vi "Set_Pulse.vi"(2 "error in":errorcluster, 3 "Data in":T1) -> (0 "error out":errorcluster, 1 "Data out":T1)   [LabVIEW 2017, in "Steps.lvlib"]
uses:
  Steps.lvlib
  Type_Defs/Data.ctl
  Type_Defs/Diagnostics.ctl
  Type_Defs/Systems.ctl
panel:
  in  "Helical Current":dbl[](array[numeric])
  in  "Toroidal Current":dbl[](array[numeric])
  in  "Time":dbl[](array[numeric])
  in  "Step Back":bool
  in  "Continue":bool
  # "Set the pulse for the next shot. Set the actual current that you want."
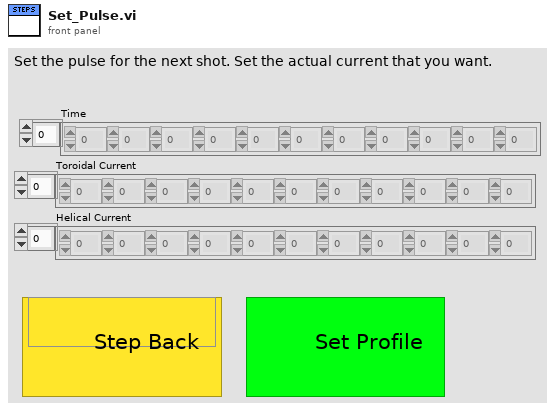
[diagram p1: front panel]
types:
  T1 = typedef "Data.ctl" = cluster{"User Name":string, "Experiment Number":i32, "Start Time":timestamp, "Data":dbl[], "Step Number":i32, "Step Instructions":string, "Diagnostics":T2, "Experiment Purpose":string, "Experiment State":enum16{"Off", "Setting Up", "Ready", "In Progress", "Shutting Down"}, "Systems":T3, "Vacuum Pressure":dbl, "Fieldpoints":cluster{"System Boolean Fieldpoints":cluster{"Compressed Air":refnum<k21>, "T-20kV Power Switch":refnum<k21>, "T-Rectifier":refnum<k21>, "Engage Interlock":refnum<k21>, "Ventilator":refnum<k21>, "Magnetron":refnum<k21>, "H-20kV Power Switch":refnum<k21>, "H-Rectifier":refnum<k21>, "Main Water Pump":refnum<k21>, "WEGA Water Pump":refnum<k21>, "Gas Inlet Valves":refnum<k21>}, "Step Fieldpoints":cluster{"Exhaust Ventillator":refnum<k21>, "Compressed Air":refnum<k21>, "Water Pressure":refnum<k21>, "Interlock":refnum<k21>, "Toroidal Power Supply 1":refnum<k21>, "Toroidal Power Supply 2":refnum<k21>, "Toroidal Rectifier":refnum<k21>, "Helical Power Supply":refnum<k21>, "Helical Rectifier":refnum<k21>, "6kW Magnetron Standby":refnum<k21>, "20kW Magnetron Standby":refnum<k21>}}, "Pressure History":cluster{"Seconds into Experiment":i32[], "Pressure Data":dbl[]}, "Time Computer Control":dbl[], "Toroidal Voltage Computer Control":dbl[], "Helical Voltage Computer Control":dbl[], "Toroidal Current":dbl[], "Toroidal Voltage":dbl[], "Toroidal Current Set Point":dbl[], "Helical Current Set Point":dbl[], "Helical Voltage":dbl[], "Helical Current":dbl[], "Experiment Folder":path, "Run Another Shot?":bool}
  T2 = typedef "Diagnostics.ctl" = cluster{"Langmuir Probe":bool, "Rogowski 1":bool, "Rogowski 2":bool, "Rogowski 3":bool, "B-dot 1":bool, "B-dot 2":bool}
  T3 = typedef "Systems.ctl" = cluster{"Compressed Air":bool, "T-20kV Power Switch":bool, "T-Rectifier":bool, "Engage Interlock":bool, "Ventilator":bool, "Magnetron":bool, "H-20kV Power Switch":bool, "H-Rectifier":bool, "Main Water Pump":bool, "WEGA Water Pump":bool, "Gas Inlet Valves":bool}
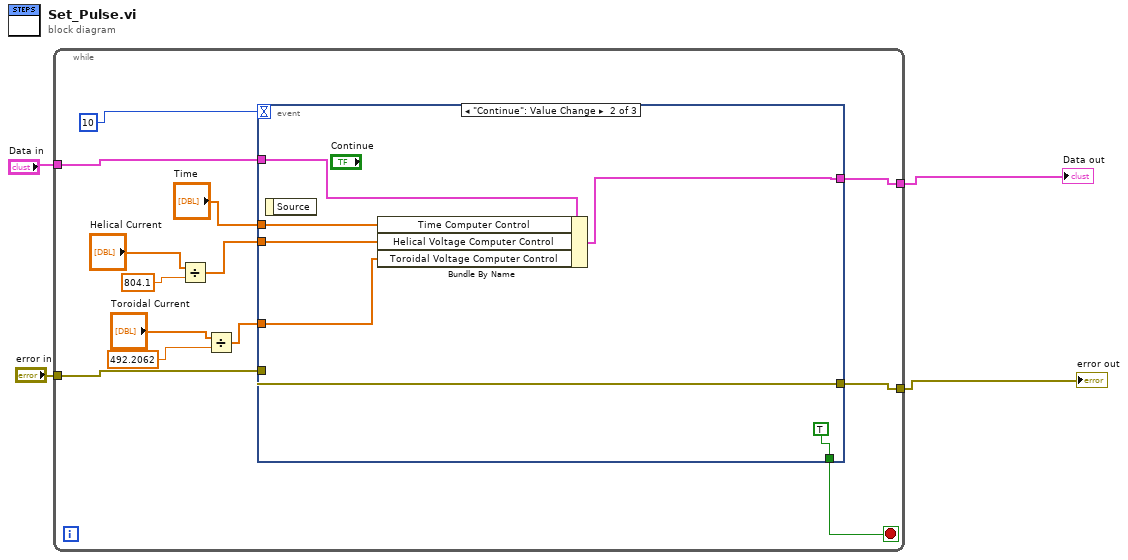
[diagram p0: block diagram]
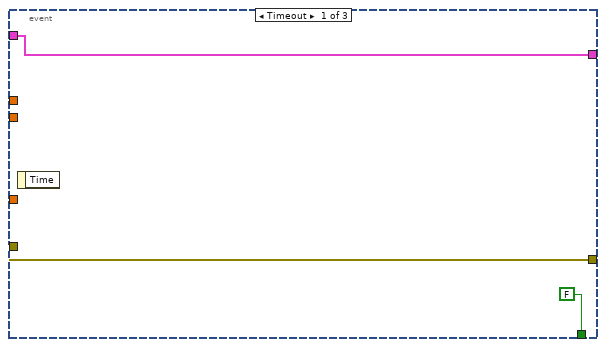
[diagram p2: hidden frame]
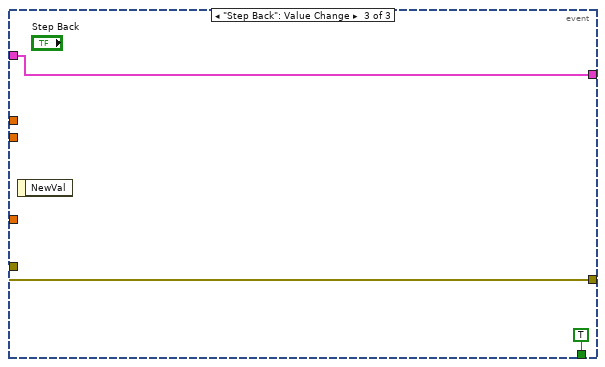
[diagram p3: hidden frame]
diagram:
  n1 = while {
    tunnel: "error in" -> [w17]
    tunnel: [w16] -> w1
    tunnel: [w14] -> w2
    tunnel: "Data in" -> [w13]
    stop <- w15 stop-if-true
    n2 = Divide(x="Helical Current", y=804.1 ("Numeric")) -> (x/y=w9:dbl[])
    n3 = Divide(x="Toroidal Current", y=492.2062 ("Numeric")) -> (x/y=w7:dbl[])
    n4 = event shown="[1] \"Continue\": Value Change" {
      selector: _ -> [_ _ _]
      dyn-events: _ -> [_ _ _]
      timeout: 10 -> [_ _ _]
      tunnel: w17 -> [w19 w27 w30]
      tunnel: [w19 w27 w30] -> w16
      tunnel: [FALSE TRUE TRUE] -> w15
      tunnel: [w18 w25 w28] -> w14
      tunnel: w13 -> [w18 w24 w28]
      tunnel: "Time" -> [_ w23 _]
      tunnel: w9 -> [_ w22 _]
      tunnel: w7 -> [_ w21 _]
      event Timeout {
        n5 = event-data() -> ()  [unwired: 1 in, 1 out]
      }
      event "Continue": Value Change {
        n6 = event-data() -> ()  [unwired: 1 in, 1 out]
        n7 = Bundle By Name(cluster=w24, "Time Computer Control"=w23, "Helical Voltage Computer Control"=w22, "Toroidal Voltage Computer Control"=w21) -> (w25:T1)
      }
      event "Step Back": Value Change {
        n8 = event-data() -> ()  [unwired: 1 in, 1 out]
      }
    }
  }
  "error out" <- w1
  "Data out" <- w2
